vi "Cannon Lock Fire.vi"(1 "Cannon Info In":T2) -> (0 "Cannon Info Out":T2)   [LabVIEW 2013]
uses:
  <vilib>/Rock Robotics/WPI/Relay/WPI_RelayValue.ctl
  <vilib>/Rock Robotics/WPI/Solenoid/WPI_SolenoidValue.ctl
  Intake/Intake Global.vi
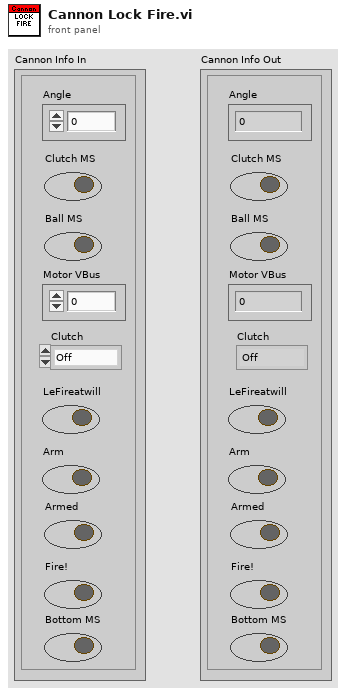
[diagram p1: front panel]
types:
  T1 = typedef "WPI_RelayValue.ctl" = enum16{"Off", "On", "Forward", "Reverse"}
  T2 = cluster{"Angle":dbl, "Clutch MS":bool, "Ball MS":bool, "Motor VBus":dbl, "Clutch ":T1, "LeFireatwill":bool, "Arm":bool, "Armed":bool, "Fire!":bool, "Bottom MS":bool}
  T3 = typedef "WPI_SolenoidValue.ctl" = enum16{"Off", "On", "Forward", "Reverse"}
  T4 = cluster{"Arm State":bool, "Gripper Out":bool, "Gripper Execution":T1, "Arm Execution":T3, "Gripper In":bool}
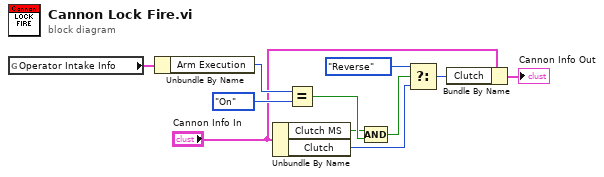
[diagram p0: block diagram]
diagram:
  n1 = global read "Intake Global.vi" "Operator Intake Info"() -> (w11:T4)
  n2 = Unbundle By Name(w11) -> ("Arm Execution"=w10:T3)
  n3 = Unbundle By Name("Cannon Info In") -> ("Clutch MS"=w1:bool, "Clutch"=w5:T1)
  n4 = Equal?(x=w10, y=WPI_SolenoidValue."On" ("Arm Execution")) -> (x = y?=w8:bool)
  n5 = Compound Arithmetic op=AND(w1, w8) -> (w4:bool)
  n6 = Select(t=WPI_SolenoidValue."Reverse" ("Arm Execution"), s=w4, f=w5) -> (s? t:f=w7:T1)
  n7 = Bundle By Name(cluster="Cannon Info In", "Clutch"=w7) -> (→"Cannon Info Out":T2)
